vi "loadDataNodeBegin.vi"(8 "error in (no error)":errorcluster, 10 "XML Refnum in":refnum<file>, 11 "DMA_Write in":refnum<class "DMA_Write.lvclass">) -> (0 "error out":errorcluster, 2 "XML Refnum out":refnum<file>, 3 "DMA_Write out":refnum<class "DMA_Write.lvclass">)   [LabVIEW 2013, in "DMA_Write.lvclass"]
doc: "Part of the file loading process. Occurs at the beginning of a node being loaded. Loads the common xceDataNode data name and description."
uses:
  DMA_Write.lvclass
  DMA_Write.lvclass/DMA_Write.ctl
  XML Parser/XML Parser.lvclass
  xCE/xceNode/xceNode.lvclass
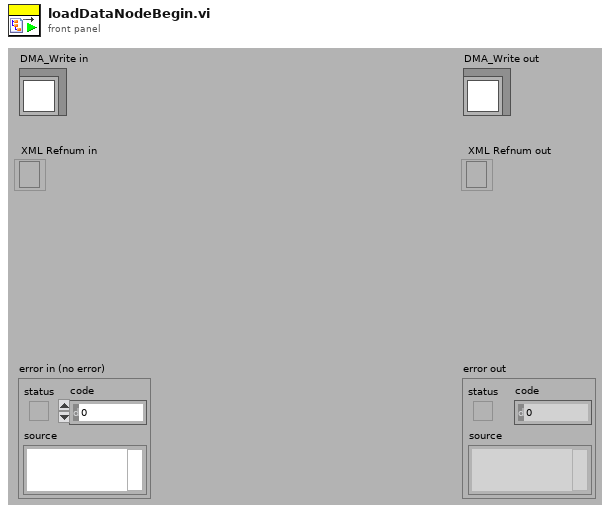
[diagram p1: front panel]
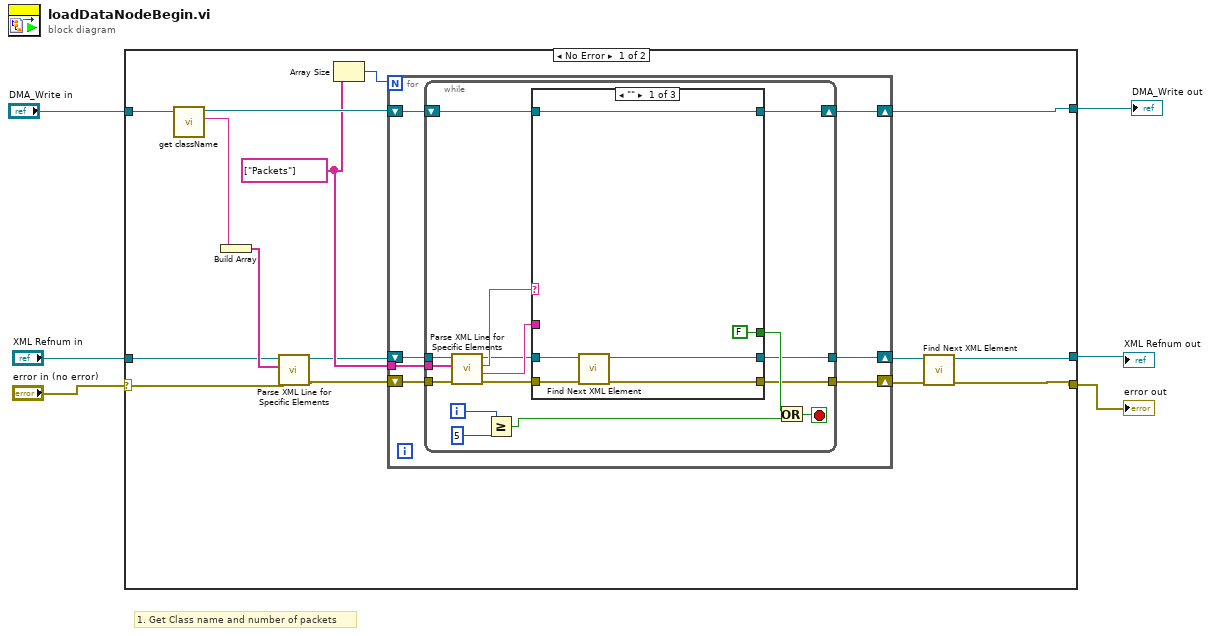
[diagram p0: block diagram]
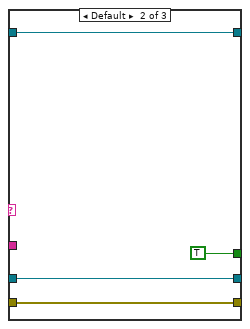
[diagram p2: hidden frame]
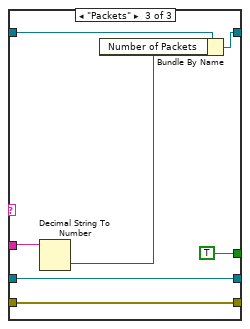
[diagram p3: hidden frame]
diagram:
  # "1. Get Class name and number of packets"
  n1 = case shown="No Error" "error in (no error)" {
    selector: "error in (no error)" -> [w11 w64]
    tunnel: [w7 w64] -> w1
    tunnel: [w20 w63] -> w3
    tunnel: [w8 w62] -> w2
    tunnel: "DMA_Write in" -> [w17 w63]
    tunnel: "XML Refnum in" -> [w12 w62]
    frame No Error {
      w15 = string[] ["Packets"] ("Token List")
      n2 = call "get className.vi"("xceNode in"=w17) -> ("Class name"=w18:string, "xceNode out"=w16:refnum<class "DMA_Write.lvclass">)  [unwired: 8 in, 1 out]
      n3 = Build Array(w18) -> (w19:string[])
      n4 = call "Parse XML Line for Specific Elements.vi"("error in (no error)"=w11, "Elements"=w19, "XML Refnum in"=w12) -> ("error out"=w13:errorcluster, "XML Refnum out"=w14:refnum<file>)  [unwired: 4 in, 3 out]
      n5 = Array Size(array=w15) -> (size(s)=w21:i32)
      n6 = for {
        N: w21 -> [_]
        tunnel: w15 -> [w28]
        shift-right: [w23] -> w20
        shift-left: w16 -> [w25]
        shift-right: [w24] -> w9
        shift-left: w14 -> [w27]
        shift-right: [w22] -> w10
        shift-left: w13 -> [w26]
        n7 = while {
          tunnel: w28 -> [w44]
          tunnel: w27 -> [w43]
          tunnel: w26 -> [w42]
          shift-right: [w37] -> w23
          shift-left: w25 -> [w39]
          tunnel: [w29] -> w24
          tunnel: [w30] -> w22
          i -> [w41]
          stop <- w34 stop-if-true
          n8 = call "Parse XML Line for Specific Elements.vi"("error in (no error)"=w42, "Elements"=w44, "XML Refnum in"=w43) -> ("error out"=w31:errorcluster, "Value"=w33:string, "Element Name"=w38:string, "XML Refnum out"=w32:refnum<file>)  [unwired: 4 in, 1 out]
          n9 = Greater Or Equal?(x=w41, y=5) -> (x >= y?=w35:bool)
          n10 = case shown="\"\"" w38 {
            tunnel: w39 -> [w50 w54 w61]
            tunnel: [w50 w54 w60] -> w37
            tunnel: [FALSE TRUE TRUE] -> w36
            tunnel: w33 -> [_ _ w56]
            tunnel: w32 -> [w48 w52 w58]
            tunnel: w31 -> [w45 w51 w57]
            tunnel: [w46 w51 w57] -> w30
            tunnel: [w47 w52 w58] -> w29
            frame "" {
              n11 = call "Find Next XML Element.vi"("error in (no error)"=w45, "XML Fine In"=w48) -> ("error out"=w46:errorcluster, "XML Fine Out"=w47:refnum<file>)  [unwired: 7 in, 1 out]
            }
            frame Default {
            }
            frame "Packets" {
              n12 = Decimal String To Number(string=w56) -> (number=w55:i32)  [unwired: 2 in, 1 out]
              n13 = Bundle By Name(cluster=w61, "Number of Packets"=w55) -> (w60:refnum<class "DMA_Write.lvclass">)
            }
          }
          n14 = Or(x=w36, y=w35) -> (x .or. y?=w34:bool)
        }
      }
      n15 = call "Find Next XML Element.vi"("error in (no error)"=w10, "XML Fine In"=w9) -> ("error out"=w7:errorcluster, "XML Fine Out"=w8:refnum<file>)  [unwired: 7 in, 1 out]
    }
    frame Error {
    }
  }
  "error out" <- w1
  "DMA_Write out" <- w3
  "XML Refnum out" <- w2
